vi "InputHeader.vi"(0 "Save Path":path, 2 "Location":T1=enum."WCM Main", 7 "Type of scan":T2, 9 "LOS Visable?":bool, 11 "TempPath":path, 12 "Array":T3(array[cluster])) -> (1 "Aborted?":bool=TRUE, 3 "Write LOS?":bool, 4 "Write Comment?":bool, 6 "Save Path Out":path, 10 "LOS":string, 14 "Use Dual Mode Folders?":bool=TRUE, 15 "Comment out":string)   [LabVIEW 2022 SP3]
uses:
  LOS.ctl
  ScanningControl/-ScanSystem/Controls/ScanType2.ctl
  ScanningControl/-ScanSystem/Controls/location.ctl
  <vilib>/Utility/miscctls.llb/LVPositionTypeDef.ctl
  <vilib>/event_ctls.llb/eventvkey.ctl
panel:
  out "Dual XDCR Folder 2":path
  in  "Use Dual Mode Folders?":bool=TRUE
  in  "Level Of Suspicion":T4
  in  "Cancel":bool
  in  "Edit Path":bool
  out "Length":i32
  in  "Header Comment":string
  in  "Save":bool
  # "Limited to 64 characters"
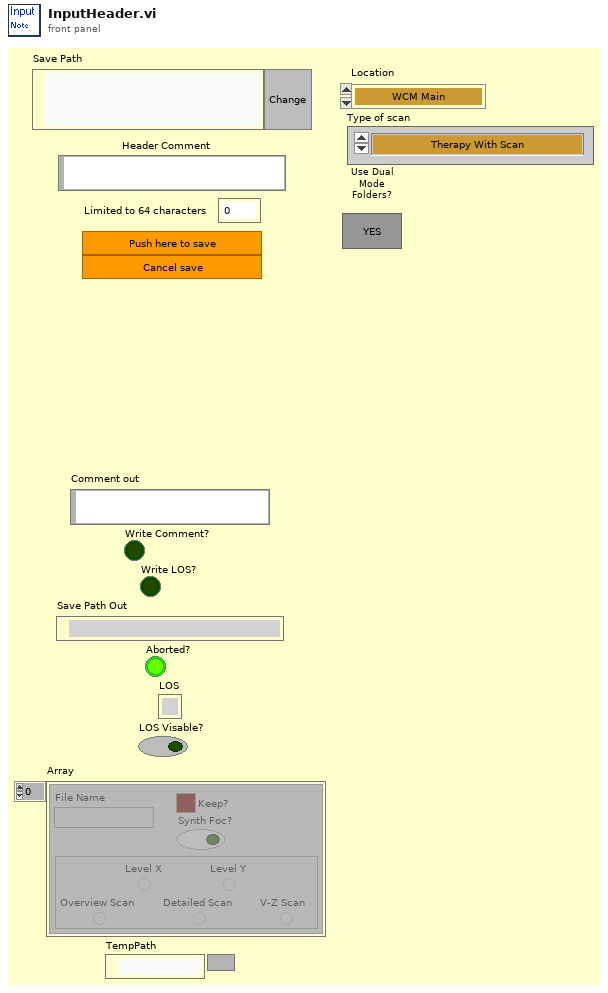
[diagram p1: front panel]
types:
  T1 = typedef "location.ctl" = enum16{"Automatic", "WCM Main", "Hawaii", "Columbia MM3000", "Columbia  NI System", "NYU", "RRI 2", "UHI Allen", "CUMC RT", "Chiba", "Stony Brook", "WCM Microscopy", "WCM Aeoretch", "WCM Optics Lab", "WCM Main 2Axis", "WCM Rotation", "WCM SAM SMAC", "SERI GP"}
  T2 = typedef "ScanType2.ctl" = enum16{"Therapy With Scan", "M scan", "M Scan With Therapy Burst", "1-D B Scan", "1-D B Scan With Therapy Burst", "2-D B Scan", "2-D B Scan With Therapy Burst", "Rotational Scan", "1-D B-Scan PRF", "2-D B-Scan PRF", "Real-Time Scan", "Contrast Agents", "1-D w/ Real-Time Set Up", "Dual Transducer", "Acoustic Microscopy", "Hydrophone Scanning"}
  T3 = cluster{"File Name":string, "Keep?":bool, "Synth Foc?":bool, "Microscopy Scan Mode":enum32{"Level X", "Level Y", "Overview Scan", "Detailed Scan", "V-Z Scan"}}[]
  T4 = typedef "LOS.ctl" = enum32{"No Selection", "1", "2", "3", "4", "5"}
  T5 = typedef "eventvkey.ctl" = enum16{"ASCII", "Enter", "Return", "Shift", "Ctrl", "Alt", "Cmd", "Opt", "Caps", "NumLock", "Clear", "Break", "Up", "Down", "Left", "Right", "Insert", "Delete", "Home", "End", "PageUp", "PageDown", "Escape", "Help", "Pause", "ScrollLock", "F1", "F2", "F3", "F4", "F5", "F6", "F7", "F8", "F9", "F10", "F11", "F12", "F13", "F14", "F15", "F16", "F17", "F18", "F19", "F20", "F21", "F22", "F23", "F24", "Play", "VolumeUp", "VolumeDown", "Mute", "Two Byte Char"}
  T6 = typedef "LVRectTypeDef.ctl" = cluster{"Left":i16, "Top":i16, "Right":i16, "Bottom":i16}
  T7 = typedef "LVPositionTypeDef.ctl" = cluster{"Left":i32, "Top":i32}
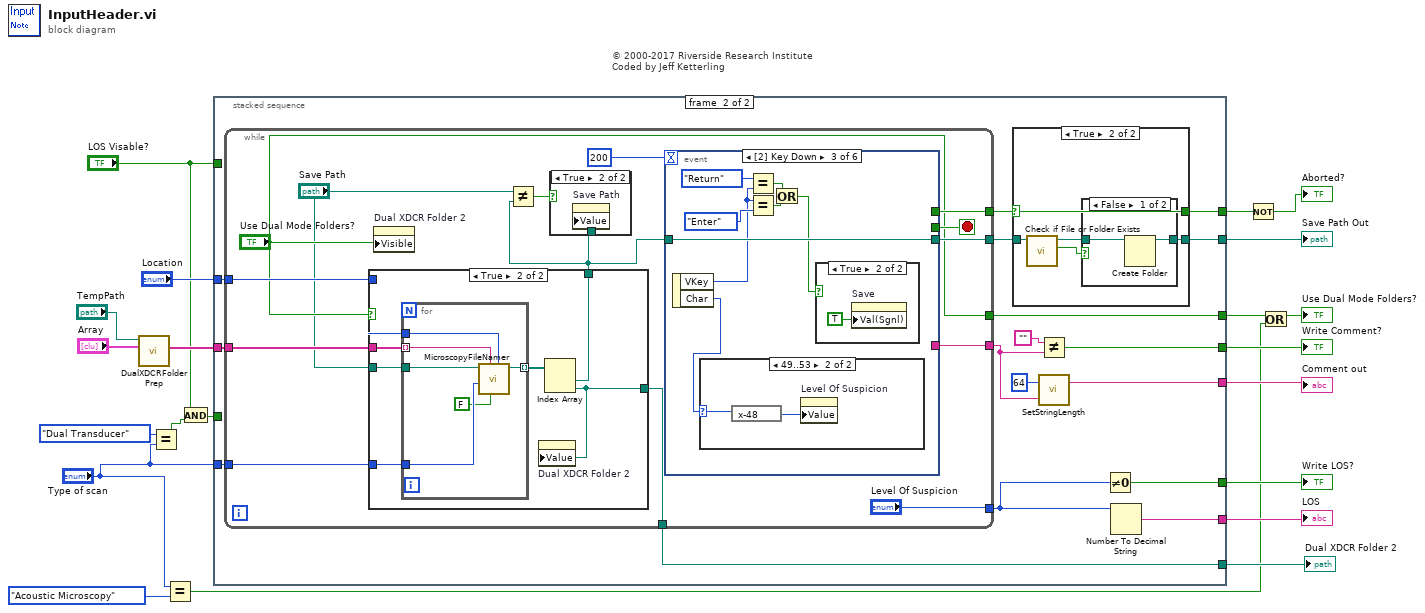
[diagram p0: block diagram]
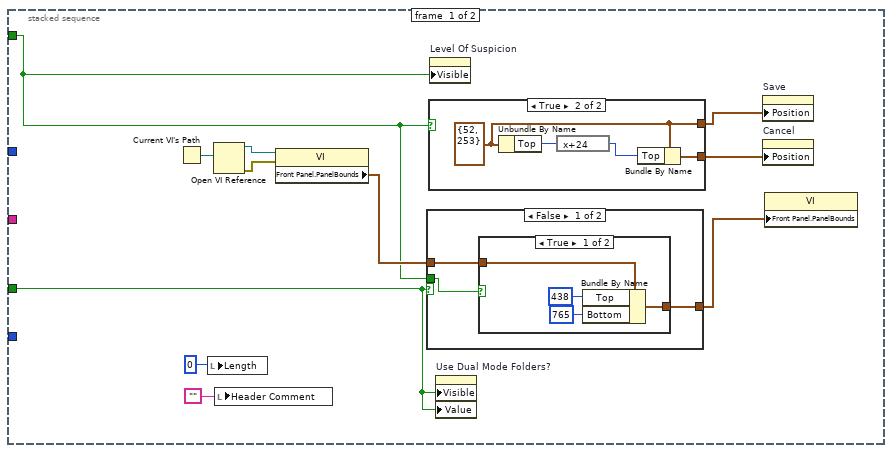
[diagram p2: hidden frame]
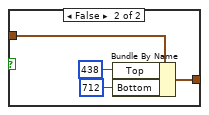
[diagram p3: hidden frame]
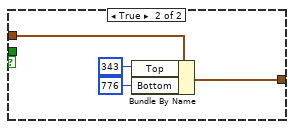
[diagram p4: hidden frame]
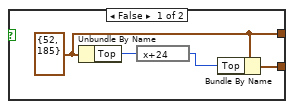
[diagram p5: hidden frame]
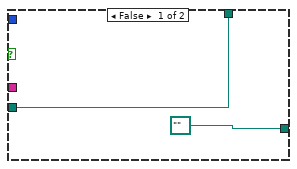
[diagram p9: hidden frame]
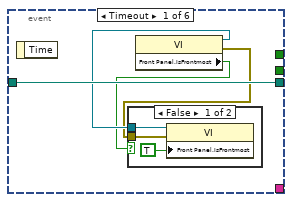
[diagram p10: hidden frame]
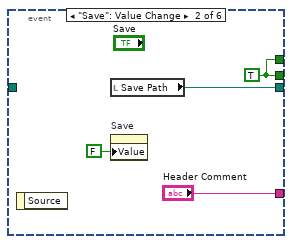
[diagram p12: hidden frame]
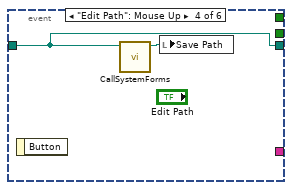
[diagram p15: hidden frame]
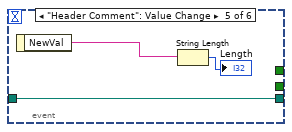
[diagram p16: hidden frame]
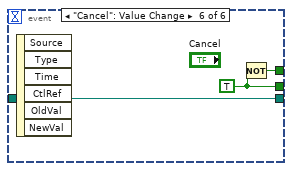
[diagram p17: hidden frame]
diagram:
  # "© 2000-2017 Riverside Research Institute\nCoded by Jeff Ketterling"
  n1 = call "DualXDCRFolderPrep.vi"("Array in"="Array", "TempPath"="TempPath") -> ("DualXdcrDataOut"=w9:string[])  [unwired: 8 in, 1 out]
  n2 = Equal?(x=ScanType2."Dual Transducer", y="Type of scan") -> (x = y?=w5:bool)
  n3 = Equal?(x="Type of scan", y=ScanType2."Acoustic Microscopy" ("x")) -> (x = y?=w3:bool)
  n4 = And(x="LOS Visable?", y=w5) -> (x .and. y?=w8:bool)
  n5 = stacked-sequence {
    tunnel: [_ w68] -> w21
    tunnel: [_ w66] -> w20
    tunnel: [_ w64] -> w18
    tunnel: [_ w63] -> w17
    tunnel: [_ w62] -> w16
    tunnel: [_ w61] -> w15
    tunnel: [_ w60] -> w14
    tunnel: w8 -> [w23 _]
    tunnel: w9 -> [_ w59]
    tunnel: "Location" -> [_ w58]
    tunnel: "Type of scan" -> [_ w57]
    tunnel: [_ w56] -> w11
    tunnel: "LOS Visable?" -> [w22 _]
    frame #0 {
      n6 = Current VI's Path() -> (path=w26:path)
      n7 = local write "Length"(0 ("Length")) -> ()
      n8 = Open VI Reference(vi path=w26) -> (vi reference=w28:refnum<vi>, error out=w27:errorcluster)  [unwired: 5 in]
      n9 = local write "Header Comment"("") -> ()
      n10 = property class="VI"(reference=w28, error in=w27) -> ("Front Panel.PanelBounds"=w25:T6)  [unwired: 2 out]
      n11 = case shown="False" w23 {
        tunnel: [w34 w46] -> w24
        tunnel: w25 -> [w35 w47]
        tunnel: w22 -> [w33 _]
        frame False {
          n12 = case shown="True" w33 {
            tunnel: w35 -> [w38 w42]
            tunnel: [w37 w41] -> w34
            frame True {
              n13 = Bundle By Name(cluster=w38, "Top"=i16 438, "Bottom"=i16 765) -> (w37:T6)
            }
            frame False {
              n14 = Bundle By Name(cluster=w42, "Top"=i16 438, "Bottom"=i16 712) -> (w41:T6)
            }
          }
        }
        frame True {
          n15 = Bundle By Name(cluster=w47, "Top"=i16 343, "Bottom"=i16 776) -> (w46:T6)
        }
      }
      n16 = case shown="True" w22 {
        tunnel: [w51 w55] -> w31
        tunnel: [w50 w54] -> w32
        frame False {
          w51 = T7 {"Left"=52, "Top"=185} ("Position")
          n17 = Unbundle By Name(w51) -> ("Top"=w49:i32)
          n18 = expression code="x+24"(w49) -> (w48:i32)
          n19 = Bundle By Name(cluster=w51, "Top"=w48) -> (w50:T7)
        }
        frame True {
          w55 = T7 {"Left"=52, "Top"=253} ("Position")
          n20 = Unbundle By Name(w55) -> ("Top"=w53:i32)
          n21 = expression code="x+24"(w53) -> (w52:i32)
          n22 = Bundle By Name(cluster=w55, "Top"=w52) -> (w54:T7)
        }
      }
      n23 = property on="Level Of Suspicion" class="RadioBtnsControl (strict)"("Visible"=w22) -> ()  [unwired: 2 in, 2 out]
      n24 = property on="Use Dual Mode Folders?" class="Bool (strict)"("Visible"=w23, "Value"=w23) -> ()  [unwired: 2 in, 2 out]
      n25 = property on="Save" class="Bool (strict)"("Position"=w31) -> ()  [unwired: 2 in, 2 out]
      n26 = property on="Cancel" class="Bool"("Position"=w32) -> ()  [unwired: 2 in, 2 out]
      n27 = property class="VI"("Front Panel.PanelBounds"=w24) -> ()  [unwired: 2 in, 2 out]
    }
    frame #1 {
      n28 = while {
        tunnel: [w94] -> w70
        tunnel: [w93] -> w69
        tunnel: [w92] -> w67
        tunnel: ["Level Of Suspicion"] -> w65
        tunnel: ["Use Dual Mode Folders?"] -> w60
        tunnel: w59 -> [w90]
        tunnel: w58 -> [w89]
        tunnel: w57 -> [w88]
        tunnel: [w87] -> w56
        stop <- w96 stop-if-true
        n29 = case shown="True" "Use Dual Mode Folders?" {
          tunnel: w90 -> [_ w105]
          tunnel: w89 -> [_ w104]
          tunnel: w88 -> [_ w103]
          tunnel: "Save Path" -> [w99 w102]
          tunnel: [path "" ("Scan Data Path") w100] -> w87
          tunnel: [w99 w101] -> w83
          frame False {
          }
          frame True {
            n30 = for {
              tunnel: w105 -> [w110] mode=indexing
              tunnel: w103 -> [w109]
              tunnel: w104 -> [w108]
              tunnel: w102 -> [w112]
              tunnel: [w111] -> w106 mode=indexing
              n31 = call "MicroscopyFileNamer.vi"("Location"=w108, "Create Folder Now?"=FALSE, "String in"=w110, "Type of scan"=w109, "Save Path In"=w112) -> ("Scan Data Path"=w111:path)  [unwired: 5 in, 1 out]
            }
            n32 = Index Array(array=w106) -> (element #1=w101:path, element #2=w100:path)  [unwired: 2 in]
            n33 = property on="Dual XDCR Folder 2" class="Path"("Value"=w100) -> ()  [unwired: 2 in, 2 out]
          }
        }
        n34 = property on="Dual XDCR Folder 2" class="Path"("Visible"="Use Dual Mode Folders?") -> ()  [unwired: 2 in, 2 out]
        n35 = Not Equal?(x="Save Path", y=w83) -> (x != y?=w85:bool)
        n36 = case shown="True" w85 {
          tunnel: w83 -> [_ w97]
          frame False {
          }
          frame True {
            n37 = property on="Save Path" class="Path"("Value"=w97) -> ()  [unwired: 2 in, 2 out]
          }
        }
        n38 = event shown="[2] Key Down" {
          selector: _ -> [_ _ _ _ _ _]
          dyn-events: _ -> [_ _ _ _ _ _]
          timeout: 200 -> [_ _ _ _ _ _]
          tunnel: [_ w121 _ _ _ w142] -> w96
          tunnel: [_ "Header Comment" _ _ _ _] -> w94
          tunnel: [w116 w122 w131 w136 w137 w140] -> w93
          tunnel: w83 -> [w116 _ w131 w136 w137 w140]
          tunnel: [_ w121 _ _ _ w141] -> w92
          event Timeout {
            n39 = event-data() -> ()  [unwired: 2 out]
            n40 = property class="VI"() -> (reference out=w115:refnum<vi>, error out=w113:errorcluster, "Front Panel.IsFrontmost"=w114:bool)  [unwired: 2 in]
            n41 = case shown="False" w114 {
              tunnel: w115 -> [w119 _]
              tunnel: w113 -> [w117 _]
              frame False {
                n42 = property class="VI"(reference=w119, error in=w117, "Front Panel.IsFrontmost"=TRUE) -> ()  [unwired: 2 out]
              }
              frame True {
              }
            }
          }
          event "Save": Value Change {
            w121 = TRUE
            n43 = event-data() -> ()  [unwired: 2 out]
            n44 = local read "Save Path"() -> (w122:path)
            n45 = property on="Save" class="Bool (strict)"("Value"=FALSE ("Save")) -> ()  [unwired: 2 in, 2 out]
          }
          event Key Down {
            n46 = event-data() -> ("VKey"=w127:T5, "Char"=w124:i16)  [unwired: 1 out]
            n47 = case shown="49..53" w124 {
              selector: w124 -> [_ w133]
              frame 0, Default {
              }
              frame 49..53 {
                n48 = expression code="x-48"(w133) -> (w132:i16)
                n49 = property on="Level Of Suspicion" class="RadioBtnsControl (strict)"("Value"=w132) -> ()  [unwired: 2 in, 2 out]
              }
            }
            n50 = Equal?(x=eventvkey."Return", y=w127) -> (x = y?=w126:bool)
            n51 = Equal?(x=w127, y=eventvkey."Enter") -> (x = y?=w130:bool)
            n52 = Or(x=w126, y=w130) -> (x .or. y?=w128:bool)
            n53 = case shown="True" w128 {
              frame False {
              }
              frame True {
                n54 = property on="Save" class="Bool (strict)"("Val(Sgnl)"=TRUE ("Value (Signaling)")) -> ()  [unwired: 2 in, 2 out]
              }
            }
          }
          event "Edit Path": Mouse Up {
            n55 = event-data() -> ()  [unwired: 2 out]
            n56 = call "CallSystemForms.vi"("Path In"=w136) -> ("Path Out"=w135:path)  [unwired: 8 in, 2 out]
            n57 = local write "Save Path"(w135) -> ()
          }
          event "Header Comment": Value Change {
            n58 = event-data() -> ("NewVal"=w138:string)  [unwired: 1 out]
            n59 = String Length(string=w138) -> (length=→"Length":i32)
          }
          event "Cancel": Value Change {
            w142 = TRUE
            n60 = event-data() -> ()  [unwired: 7 out]
            n61 = Not(x=w142) -> (.not. x?=w141:bool)
          }
        }
      }
      n62 = case shown="True" w67 {
        selector: w67 -> [w73 w75]
        tunnel: w69 -> [w74 w79]
        tunnel: [w74 w78] -> w68
        tunnel: [w73 w75] -> w66
        frame False {
        }
        frame True {
          n63 = call <vilib>:"Check if File or Folder Exists.vi"("path"=w79) -> ("file or folder exists?"=w76:bool, "dup path"=w77:path)  [unwired: 8 in, 1 out]
          n64 = case shown="False" w76 {
            tunnel: [w81 w82] -> w78
            tunnel: w77 -> [w80 w82]
            frame False {
              n65 = Create Folder(path (use dialog)=w80) -> (created path=w81:path)  [unwired: 2 in, 2 out]
            }
            frame True {
            }
          }
        }
      }
      n66 = Not Equal?(x="", y=w70) -> (x != y?=w64:bool)
      n67 = call "SetStringLength.vi"("Input String"=w70, "String Length"=64) -> ("Output String"=w62:string)  [unwired: 1 out]
      n68 = Not Equal To 0?(x=w65) -> (x != 0?=w63:bool)
      n69 = Number To Decimal String(number=w65) -> (decimal integer string=w61:string)  [unwired: 1 in]
    }
  }
  "Write Comment?" <- w18
  "Save Path Out" <- w21
  "Write LOS?" <- w17
  "Comment out" <- w16
  "LOS" <- w15
  "Dual XDCR Folder 2" <- w11
  n70 = Not(x=w20) -> (.not. x?=→"Aborted?":bool)
  n71 = Or(x=w14, y=w3) -> (x .or. y?=→"Use Dual Mode Folders?":bool)
